vi "Inject VI.vi"(0 "VISA Rescource name":refnum<visa-resource-name>, 1 "Delay before going back to load position (ms)":u32=500 min=500 max=5000) -> ()   [LabVIEW 2018]
uses:
  <vilib>/Instr/_visa.llb/VISA Configure Serial Port (Instr).vi
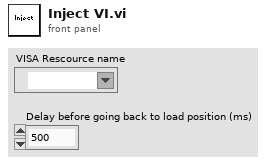
[diagram p1: front panel]
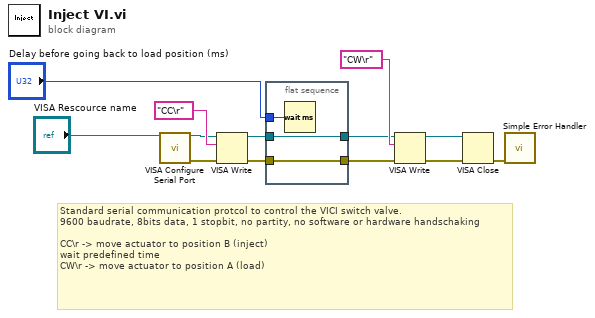
[diagram p0: block diagram]
diagram:
  # "Standard serial communication protcol to control the VICI switch valve. \n9600 baudrate, 8bits data, 1 stopbit, no partity, no software or hardware handschaking\n\nCC\\r -> move actuator to position B (inject)\nwait predefined time\nCW\\r -> move actuator to position A (load)"
  n1 = call-poly "VISA Configure Serial Port"("VISA resource name"="VISA Rescource name") -> ("VISA resource name out"=w3:refnum<visa-resource-name>, "error out"=w2:errorcluster)  [unwired: 8 in, 5 out]
  n2 = VISA Write(VISA resource name=w3, write buffer="CC\r" ("Command"), error in (no error)=w2) -> (VISA resource name out=w5:refnum<visa-resource-name>, error out=w4:errorcluster)  [unwired: 1 out]
  n3 = flat-sequence {
    tunnel: w4 -> [w15]
    tunnel: [w15] -> w9
    tunnel: w5 -> [w14]
    tunnel: [w14] -> w8
    tunnel: "Delay before going back to load position (ms)" -> [w16]
    frame #0 {
      n4 = Wait (ms)(milliseconds to wait=w16) -> ()  [unwired: 1 out]
    }
  }
  n5 = VISA Write(VISA resource name=w8, write buffer="CW\r" ("Command"), error in (no error)=w9) -> (VISA resource name out=w12:refnum<visa-resource-name>, error out=w10:errorcluster)  [unwired: 1 out]
  n6 = VISA Close(VISA resource name=w12, error in (no error)=w10) -> (error out=w11:errorcluster)
  n7 = call <vilib>:"Simple Error Handler.vi"("error in (no error)"=w11) -> ()  [unwired: 1 in, 8 out]
